vi "Check__SPath changed_IPath unchanged.vi"(9 "Current Image Pixels":cluster{"X Pixels":i32, "Y Pixels":i32}, 10 "Calibration Type":string, 11 "configuration file path":path) -> (3 "Keys with S_Path change (and I_Path unchanged)":string[](array[string]))   [LabVIEW 2012]
uses:
  Custom Controls and Typedefs/FGV_CalibrationKeyParams_Actions.ctl
  <vilib>/Utility/config.llb/NI_LVConfig.lvlib
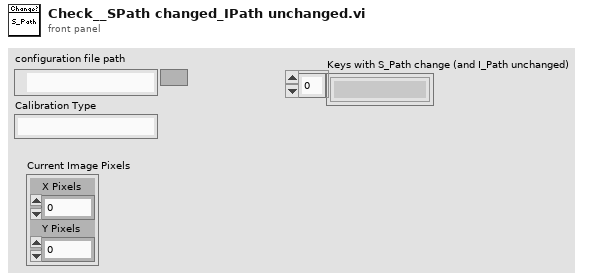
[diagram p1: front panel]
types:
  T1 = typedef "NI_LVConfig.lvlib/Config Data RefNum.ctl" = refnum<k1>
  T2 = typedef "FGV_CalibrationKeyParams_Actions.ctl" = enum16{"Initialize", "Grab From SciScan and Store", "Read Parameters", "ReadGFGValue"}
  T3 = typedef "Calibration Key Param structure.ctl" = cluster{"GFG Variable Name":string, "Data Type":T4, "Value":variant}
  T4 = typedef "VariantType.lvlib/Type.ctl" = enum8{"Invalid Type", "Void", "I8", "I16", "I32", "I64", "U8", "U16", "U32", "U64", "Single Float", "Double Float", "Extended Float", "Single Complex", "Double Complex", "Extended Complex", "Enum U8", "Enum U16", "Enum U32", "Enum U64", "Single Float With Unit", "Double Float With Unit", "Extended Float With Unit", "Single Complex with Unit", "Double Complex with Unit", "Extended Complex with Unit", "Boolean", "String", "Path", "Picture", "Tag", "Array", "Cluster", "Variant", "LV Variant", "Waveform", "Timestamp", "Digital Waveform", "Digital Data", "ExpressData", "Refnum", "External Data", "VI", "Poly VI", "LabVIEW Class Instance", "Fixed Point"}
  T5 = cluster{"Key Parameters Array":T3[], "Key String":string}
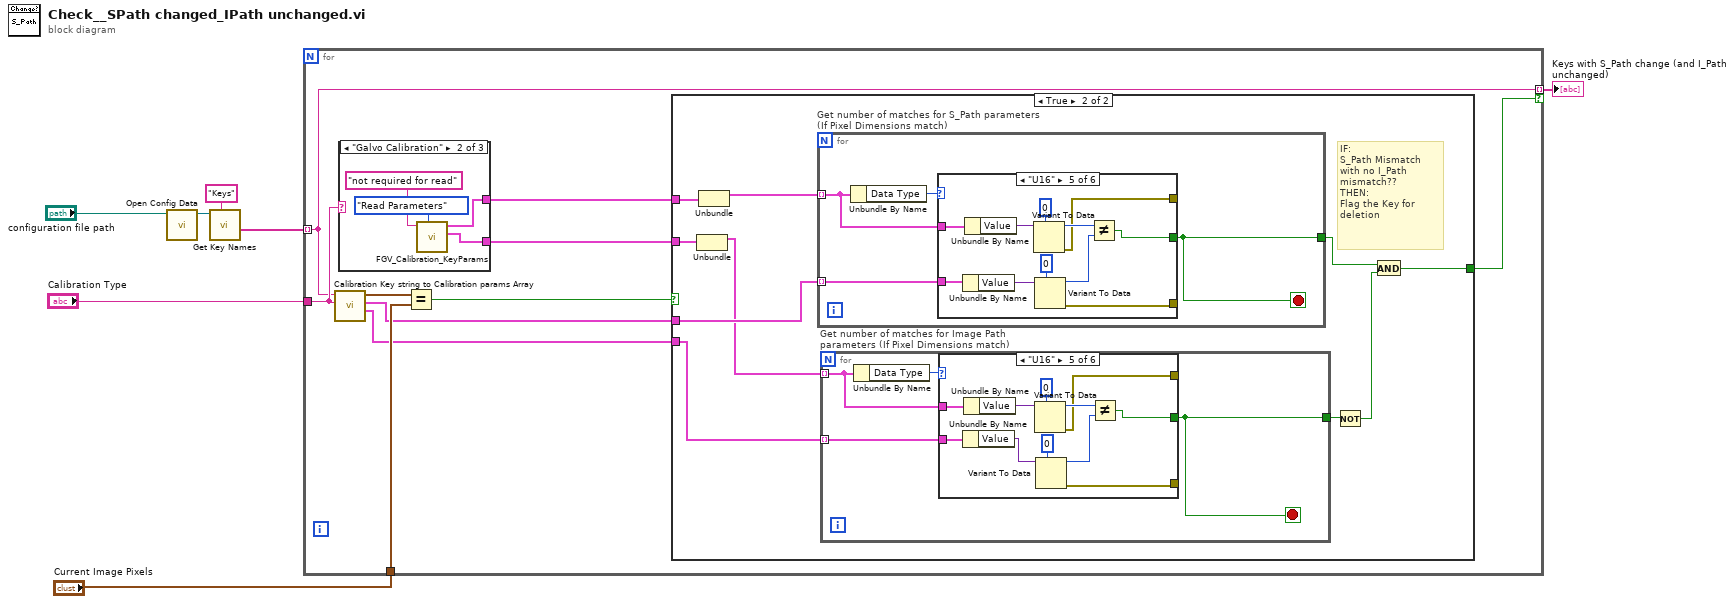
[diagram p0: block diagram]
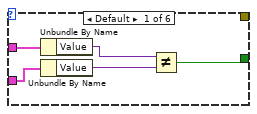
[diagram p3: hidden frame]
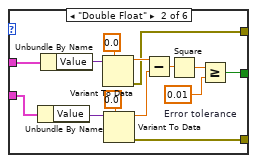
[diagram p4: hidden frame]
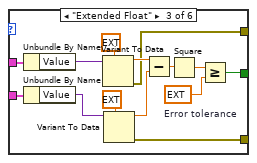
[diagram p5: hidden frame]
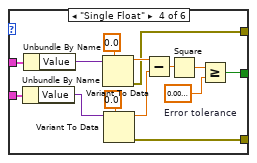
[diagram p6: hidden frame]
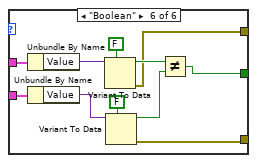
[diagram p7: hidden frame]
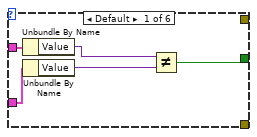
[diagram p8: hidden frame]
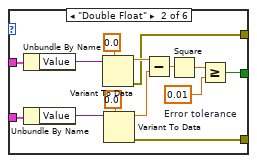
[diagram p9: hidden frame]
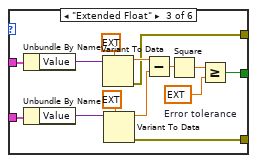
[diagram p10: hidden frame]
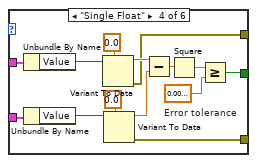
[diagram p11: hidden frame]
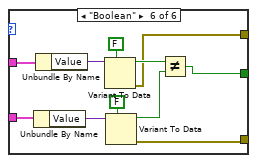
[diagram p12: hidden frame]
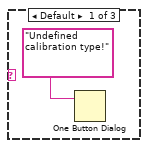
[diagram p13: hidden frame]
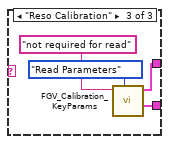
[diagram p14: hidden frame]
diagram:
  n1 = call <vilib>:"Open Config Data.vi"("configuration file path"="configuration file path") -> ("refnum"=w6:T1)  [unwired: 8 in, 2 out]
  n2 = call <vilib>:"Get Key Names.vi"("section"="Keys", "refnum"=w6) -> ("key names"=w5:string[])  [unwired: 6 in, 3 out]
  n3 = for {
    tunnel: w5 -> [w9] mode=indexing
    tunnel: "Calibration Type" -> [w17]
    tunnel: "Current Image Pixels" -> [w15]
    tunnel: [w9] -> w1 mode=indexing if=w8
    n4 = call "Calibration Key string to Calibration params Array.vi"("Calibration Type"=w17, "Key String IN"=w9) -> ("Imaging (Galvo/Reso) Key Array"=w12:T3[], "Photostim Galvo Key Array"=w13:T3[], "Image Pixels OUT"=w16:cluster{"X Pixels":i32, "Y Pixels":i32})  [unwired: 7 in]
    n5 = case shown="\"Galvo Calibration\"" w17 {
      tunnel: [_ w176 w180] -> w11
      tunnel: [_ w175 w179] -> w10
      frame Default {
        n6 = One Button Dialog(message="Undefined calibration type!") -> ()  [unwired: 1 in, 1 out]
      }
      frame "Galvo Calibration" {
        n7 = call "FGV_Calibration_KeyParams.vi"("Action"=FGV_CalibrationKeyParams_Actions."Read Parameters", "System Type"="not required for read") -> ("Imaging Galvo Key Parameters"=w175:T5, "Stimulating Galvo Key Parameters"=w176:T5)  [unwired: 4 in, 4 out]
      }
      frame "Reso Calibration" {
        n8 = call "FGV_Calibration_KeyParams.vi"("Action"=FGV_CalibrationKeyParams_Actions."Read Parameters", "System Type"="not required for read") -> ("Imaging Reso Key Parameters"=w179:T5, "Stimulating Galvo Key Parameters"=w180:T5)  [unwired: 4 in, 4 out]
      }
    }
    n9 = Equal?(x=w16, y=w15) -> (x = y?=w14:bool)
    n10 = case shown="True" w14 {
      tunnel: w13 -> [_ w24]
      tunnel: w12 -> [_ w22]
      tunnel: w11 -> [_ w27]
      tunnel: w10 -> [_ w26]
      tunnel: [_ w18] -> w8
      frame False {
      }
      frame True {
        # "IF:\nS_Path Mismatch with no I_Path mismatch??\nTHEN:\nFlag the Key for deletion"
        n11 = Unbundle(w26) -> ("Key Parameters Array"=w23:T3[])  [unwired: 1 out]
        n12 = Unbundle(w27) -> ("Key Parameters Array"=w25:T3[])  [unwired: 1 out]
        n13 = for "Get number of matches for S_Path parameters (If Pixel Dimensions match)" {
          tunnel: w25 -> [w103] mode=indexing
          tunnel: w24 -> [w102] mode=indexing
          tunnel: [w101] -> w20
          stop <- w101 stop-if-true
          n14 = Unbundle By Name(w103) -> ("Data Type"=w104:T4)
          n15 = case shown="\"U16\"" w104 {
            tunnel: w102 -> [w109 w122 w136 w150 w161 w172]
            tunnel: [w106 w112 w126 w140 w154 w167] -> w101
            tunnel: w103 -> [w105 w123 w137 w151 w162 w173]
            tunnel: [_ w111 w124 w139 w153 w164] -> _
            tunnel: [_ w110 w125 w138 w152 w163] -> _
            frame Default {
              n16 = Unbundle By Name(w105) -> ("Value"=w108:variant)
              n17 = Unbundle By Name(w109) -> ("Value"=w107:variant)
              n18 = Not Equal?(x=w108, y=w107) -> (x != y?=w106:bool)
            }
            frame "Double Float" {
              w114 = 0.01  # Error tolerance
              n19 = Unbundle By Name(w123) -> ("Value"=w121:variant)
              n20 = Unbundle By Name(w122) -> ("Value"=w118:variant)
              n21 = Variant To Data(type=0.0, Variant=w121) -> (data=w117:dbl, error out=w111:errorcluster)  [unwired: 1 in]
              n22 = Variant To Data(type=0.0, Variant=w118) -> (data=w116:dbl, error out=w110:errorcluster)  [unwired: 1 in]
              n23 = Subtract(x=w117, y=w116) -> (x-y=w115:dbl)
              n24 = Square(x=w115) -> (x^2=w113:dbl)
              n25 = Greater Or Equal?(x=w113, y=w114) -> (x >= y?=w112:bool)
            }
            frame "Extended Float" {
              w128 = ext 0.01  # Error tolerance
              n26 = Unbundle By Name(w137) -> ("Value"=w135:variant)
              n27 = Unbundle By Name(w136) -> ("Value"=w132:variant)
              n28 = Variant To Data(type=ext 0.0, Variant=w135) -> (data=w131:ext, error out=w124:errorcluster)  [unwired: 1 in]
              n29 = Variant To Data(type=ext 0.0, Variant=w132) -> (data=w130:ext, error out=w125:errorcluster)  [unwired: 1 in]
              n30 = Subtract(x=w131, y=w130) -> (x-y=w129:ext)
              n31 = Square(x=w129) -> (x^2=w127:ext)
              n32 = Greater Or Equal?(x=w127, y=w128) -> (x >= y?=w126:bool)
            }
            frame "Single Float" {
              w142 = sgl 0.01  # Error tolerance
              n33 = Unbundle By Name(w151) -> ("Value"=w149:variant)
              n34 = Unbundle By Name(w150) -> ("Value"=w146:variant)
              n35 = Variant To Data(type=sgl 0.0, Variant=w149) -> (data=w145:sgl, error out=w139:errorcluster)  [unwired: 1 in]
              n36 = Variant To Data(type=sgl 0.0, Variant=w146) -> (data=w144:sgl, error out=w138:errorcluster)  [unwired: 1 in]
              n37 = Subtract(x=w145, y=w144) -> (x-y=w143:sgl)
              n38 = Square(x=w143) -> (x^2=w141:sgl)
              n39 = Greater Or Equal?(x=w141, y=w142) -> (x >= y?=w140:bool)
            }
            frame "U16" {
              n40 = Unbundle By Name(w161) -> ("Value"=w157:variant)
              n41 = Unbundle By Name(w162) -> ("Value"=w159:variant)
              n42 = Variant To Data(type=u16 0, Variant=w159) -> (data=w156:u16, error out=w153:errorcluster)  [unwired: 1 in]
              n43 = Variant To Data(type=u16 0, Variant=w157) -> (data=w155:u16, error out=w152:errorcluster)  [unwired: 1 in]
              n44 = Not Equal?(x=w156, y=w155) -> (x != y?=w154:bool)
            }
            frame "Boolean" {
              n45 = Unbundle By Name(w172) -> ("Value"=w170:variant)
              n46 = Unbundle By Name(w173) -> ("Value"=w171:variant)
              n47 = Variant To Data(type=FALSE, Variant=w171) -> (data=w169:bool, error out=w164:errorcluster)  [unwired: 1 in]
              n48 = Variant To Data(type=FALSE, Variant=w170) -> (data=w168:bool, error out=w163:errorcluster)  [unwired: 1 in]
              n49 = Not Equal?(x=w169, y=w168) -> (x != y?=w167:bool)
            }
          }
        }
        n50 = for "Get number of matches for Image Path parameters (If Pixel Dimensions match)" {
          tunnel: w23 -> [w30] mode=indexing
          tunnel: w22 -> [w29] mode=indexing
          tunnel: [w28] -> w21
          stop <- w28 stop-if-true
          n51 = Unbundle By Name(w30) -> ("Data Type"=w31:T4)
          n52 = case shown="\"U16\"" w31 {
            tunnel: [w34 w40 w54 w68 w82 w95] -> w28
            tunnel: w30 -> [w33 w50 w64 w78 w89 w100]
            tunnel: w29 -> [w32 w39 w53 w67 w81 w92]
            tunnel: [_ w38 w51 w66 w80 w91] -> _
            tunnel: [_ w37 w52 w65 w79 w90] -> _
            frame Default {
              n53 = Unbundle By Name(w33) -> ("Value"=w36:variant)
              n54 = Unbundle By Name(w32) -> ("Value"=w35:variant)
              n55 = Not Equal?(x=w36, y=w35) -> (x != y?=w34:bool)
            }
            frame "Double Float" {
              w42 = 0.01  # Error tolerance
              n56 = Unbundle By Name(w39) -> ("Value"=w46:variant)
              n57 = Unbundle By Name(w50) -> ("Value"=w49:variant)
              n58 = Variant To Data(type=0.0, Variant=w49) -> (data=w45:dbl, error out=w38:errorcluster)  [unwired: 1 in]
              n59 = Variant To Data(type=0.0, Variant=w46) -> (data=w44:dbl, error out=w37:errorcluster)  [unwired: 1 in]
              n60 = Subtract(x=w45, y=w44) -> (x-y=w43:dbl)
              n61 = Square(x=w43) -> (x^2=w41:dbl)
              n62 = Greater Or Equal?(x=w41, y=w42) -> (x >= y?=w40:bool)
            }
            frame "Extended Float" {
              w56 = ext 0.01  # Error tolerance
              n63 = Unbundle By Name(w64) -> ("Value"=w63:variant)
              n64 = Unbundle By Name(w53) -> ("Value"=w60:variant)
              n65 = Variant To Data(type=ext 0.0, Variant=w63) -> (data=w59:ext, error out=w51:errorcluster)  [unwired: 1 in]
              n66 = Variant To Data(type=ext 0.0, Variant=w60) -> (data=w58:ext, error out=w52:errorcluster)  [unwired: 1 in]
              n67 = Subtract(x=w59, y=w58) -> (x-y=w57:ext)
              n68 = Square(x=w57) -> (x^2=w55:ext)
              n69 = Greater Or Equal?(x=w55, y=w56) -> (x >= y?=w54:bool)
            }
            frame "Single Float" {
              w70 = sgl 0.01  # Error tolerance
              n70 = Unbundle By Name(w67) -> ("Value"=w74:variant)
              n71 = Unbundle By Name(w78) -> ("Value"=w77:variant)
              n72 = Variant To Data(type=sgl 0.0, Variant=w77) -> (data=w73:sgl, error out=w66:errorcluster)  [unwired: 1 in]
              n73 = Variant To Data(type=sgl 0.0, Variant=w74) -> (data=w72:sgl, error out=w65:errorcluster)  [unwired: 1 in]
              n74 = Subtract(x=w73, y=w72) -> (x-y=w71:sgl)
              n75 = Square(x=w71) -> (x^2=w69:sgl)
              n76 = Greater Or Equal?(x=w69, y=w70) -> (x >= y?=w68:bool)
            }
            frame "U16" {
              n77 = Unbundle By Name(w81) -> ("Value"=w85:variant)
              n78 = Unbundle By Name(w89) -> ("Value"=w87:variant)
              n79 = Variant To Data(type=u16 0, Variant=w87) -> (data=w84:u16, error out=w80:errorcluster)  [unwired: 1 in]
              n80 = Variant To Data(type=u16 0, Variant=w85) -> (data=w83:u16, error out=w79:errorcluster)  [unwired: 1 in]
              n81 = Not Equal?(x=w84, y=w83) -> (x != y?=w82:bool)
            }
            frame "Boolean" {
              n82 = Unbundle By Name(w100) -> ("Value"=w99:variant)
              n83 = Unbundle By Name(w92) -> ("Value"=w98:variant)
              n84 = Variant To Data(type=FALSE, Variant=w99) -> (data=w97:bool, error out=w91:errorcluster)  [unwired: 1 in]
              n85 = Variant To Data(type=FALSE, Variant=w98) -> (data=w96:bool, error out=w90:errorcluster)  [unwired: 1 in]
              n86 = Not Equal?(x=w97, y=w96) -> (x != y?=w95:bool)
            }
          }
        }
        n87 = Not(x=w21) -> (.not. x?=w19:bool)
        n88 = And(x=w20, y=w19) -> (x .and. y?=w18:bool)
      }
    }
  }
  "Keys with S_Path change (and I_Path unchanged)" <- w1
